vi "一体站流程自动启动.vi"(11 "参数":T1) -> ()   [LabVIEW 2016, in "PLC.lvlib"]
uses:
  PLC.lvlib
panel:
  out "s? t:f":enum16{"初始化", "采配水启动", "仪器操作", "反冲洗", "结束"}(ring)
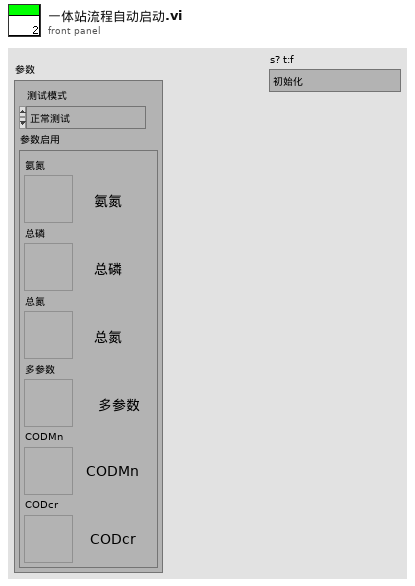
[diagram p1: front panel]
types:
  T1 = cluster{"测试模式":enum16{"正常测试", "集成干预"}, "参数启用":cluster{"氨氮":bool, "总磷":bool, "总氮":bool, "多参数":bool, "CODMn":bool, "CODcr":bool}}
  T2 = cluster{"命令":string, cluster{"starting address":u16, "holding register value":u16}}
  T3 = enum16{"启动测量", "标样核查", "零点核查", "跨度核查", "空白测试", "平行样测试", "加标回收", "空白校准", "标样校准", "初始化（清洗）", "停止测试", "仪器重启", "校时", "模式设置", "测量间隔设置"}
  T4 = cluster{"时间标识":timestamp, "设备":string, "日志信息":string, "流程参数":string}
  T5 = cluster{"测量模式":enum16{"水样测量", "标样核查", "零点核查", "跨度核查", "空白测试", "加标回收", "平行样", "校零", "校标"}}
  T6 = cluster{"时间标识":timestamp, "设备":string, "日志信息":string}
  T7 = enum16{"空闲", "水样测试", "标样核查", "零点核查", "跨度核查", "空白测试", "平行样测试", "加标回收", "空白校准", "标样校准", "初始化（清洗）"}
  T8 = cluster{"R0":i16, "R1":i16, "R2":i16, "R3":i16, "R4":i16, "R5":i16, "R6":i16, "R7":i16, "R8":i16, "R9":i16, "R10":i16, "R11":i16, "R12":i16, "R13":i16, "R14":i16, "R15":i16, "R16":i16, "R17":i16, "R18":i16, "R19":i16, "R20":i16, "R21":i16, "R22":i16, "R23":i16, "R24":i16, "R25":i16, "R26":i16, "R27":i16, "R28":i16, "R29":i16, "R30":i16, "R31":i16, "R32":i16, "R33":i16, "R34":i16, "R35":i16, "R36":i16, "R37":i16, "R38":i16, "R39":i16, "R40":i16, "R41":i16, "R42":i16, "R43":i16, "R44":i16, "R45":i16, "R46":i16, "R47":i16, "R48":i16, "R49":i16, "R50":i16, "R51":i16, "R52":i16, "R53":i16, "R54":i16, "R55":i16, "R56":i16}
  T9 = cluster{"R100":i16, "R101":i16, "R102":i16, "R103":i16, "R104":i16, "R105":i16, "R106":i16, "R107":i16, "R108":i16, "R109":i16, "R110":i16, "R111":i16, "R112":i16, "R113":i16, "R114":i16, "R115":i16, "R116":i16, "R117":i16, "R118":i16, "R119":i16, "R120":i16, "R121":i16, "R122":i16, "R123":i16}
  T10 = enum32{"Bad", "Idle", "Run top level", "Running"}
  T11 = cluster{"水样测试量程模式":enum16{"H", "L", "AUTO"}, "空白核查量程模式":enum16{"H", "L", "AUTO"}, "跨度核查量程模式":enum16{"H", "L", "AUTO"}}
  T12 = cluster{"氨氮":bool, "总磷":bool, "总氮":bool, "多参数":bool, "CODMn":bool, "CODcr":bool}
  T13 = cluster{"时间标识":timestamp, "参数":string, "集成干预测试浓度值":dbl, "集成干预前测试时间":timestamp, "集成干预前测试浓度值":dbl}
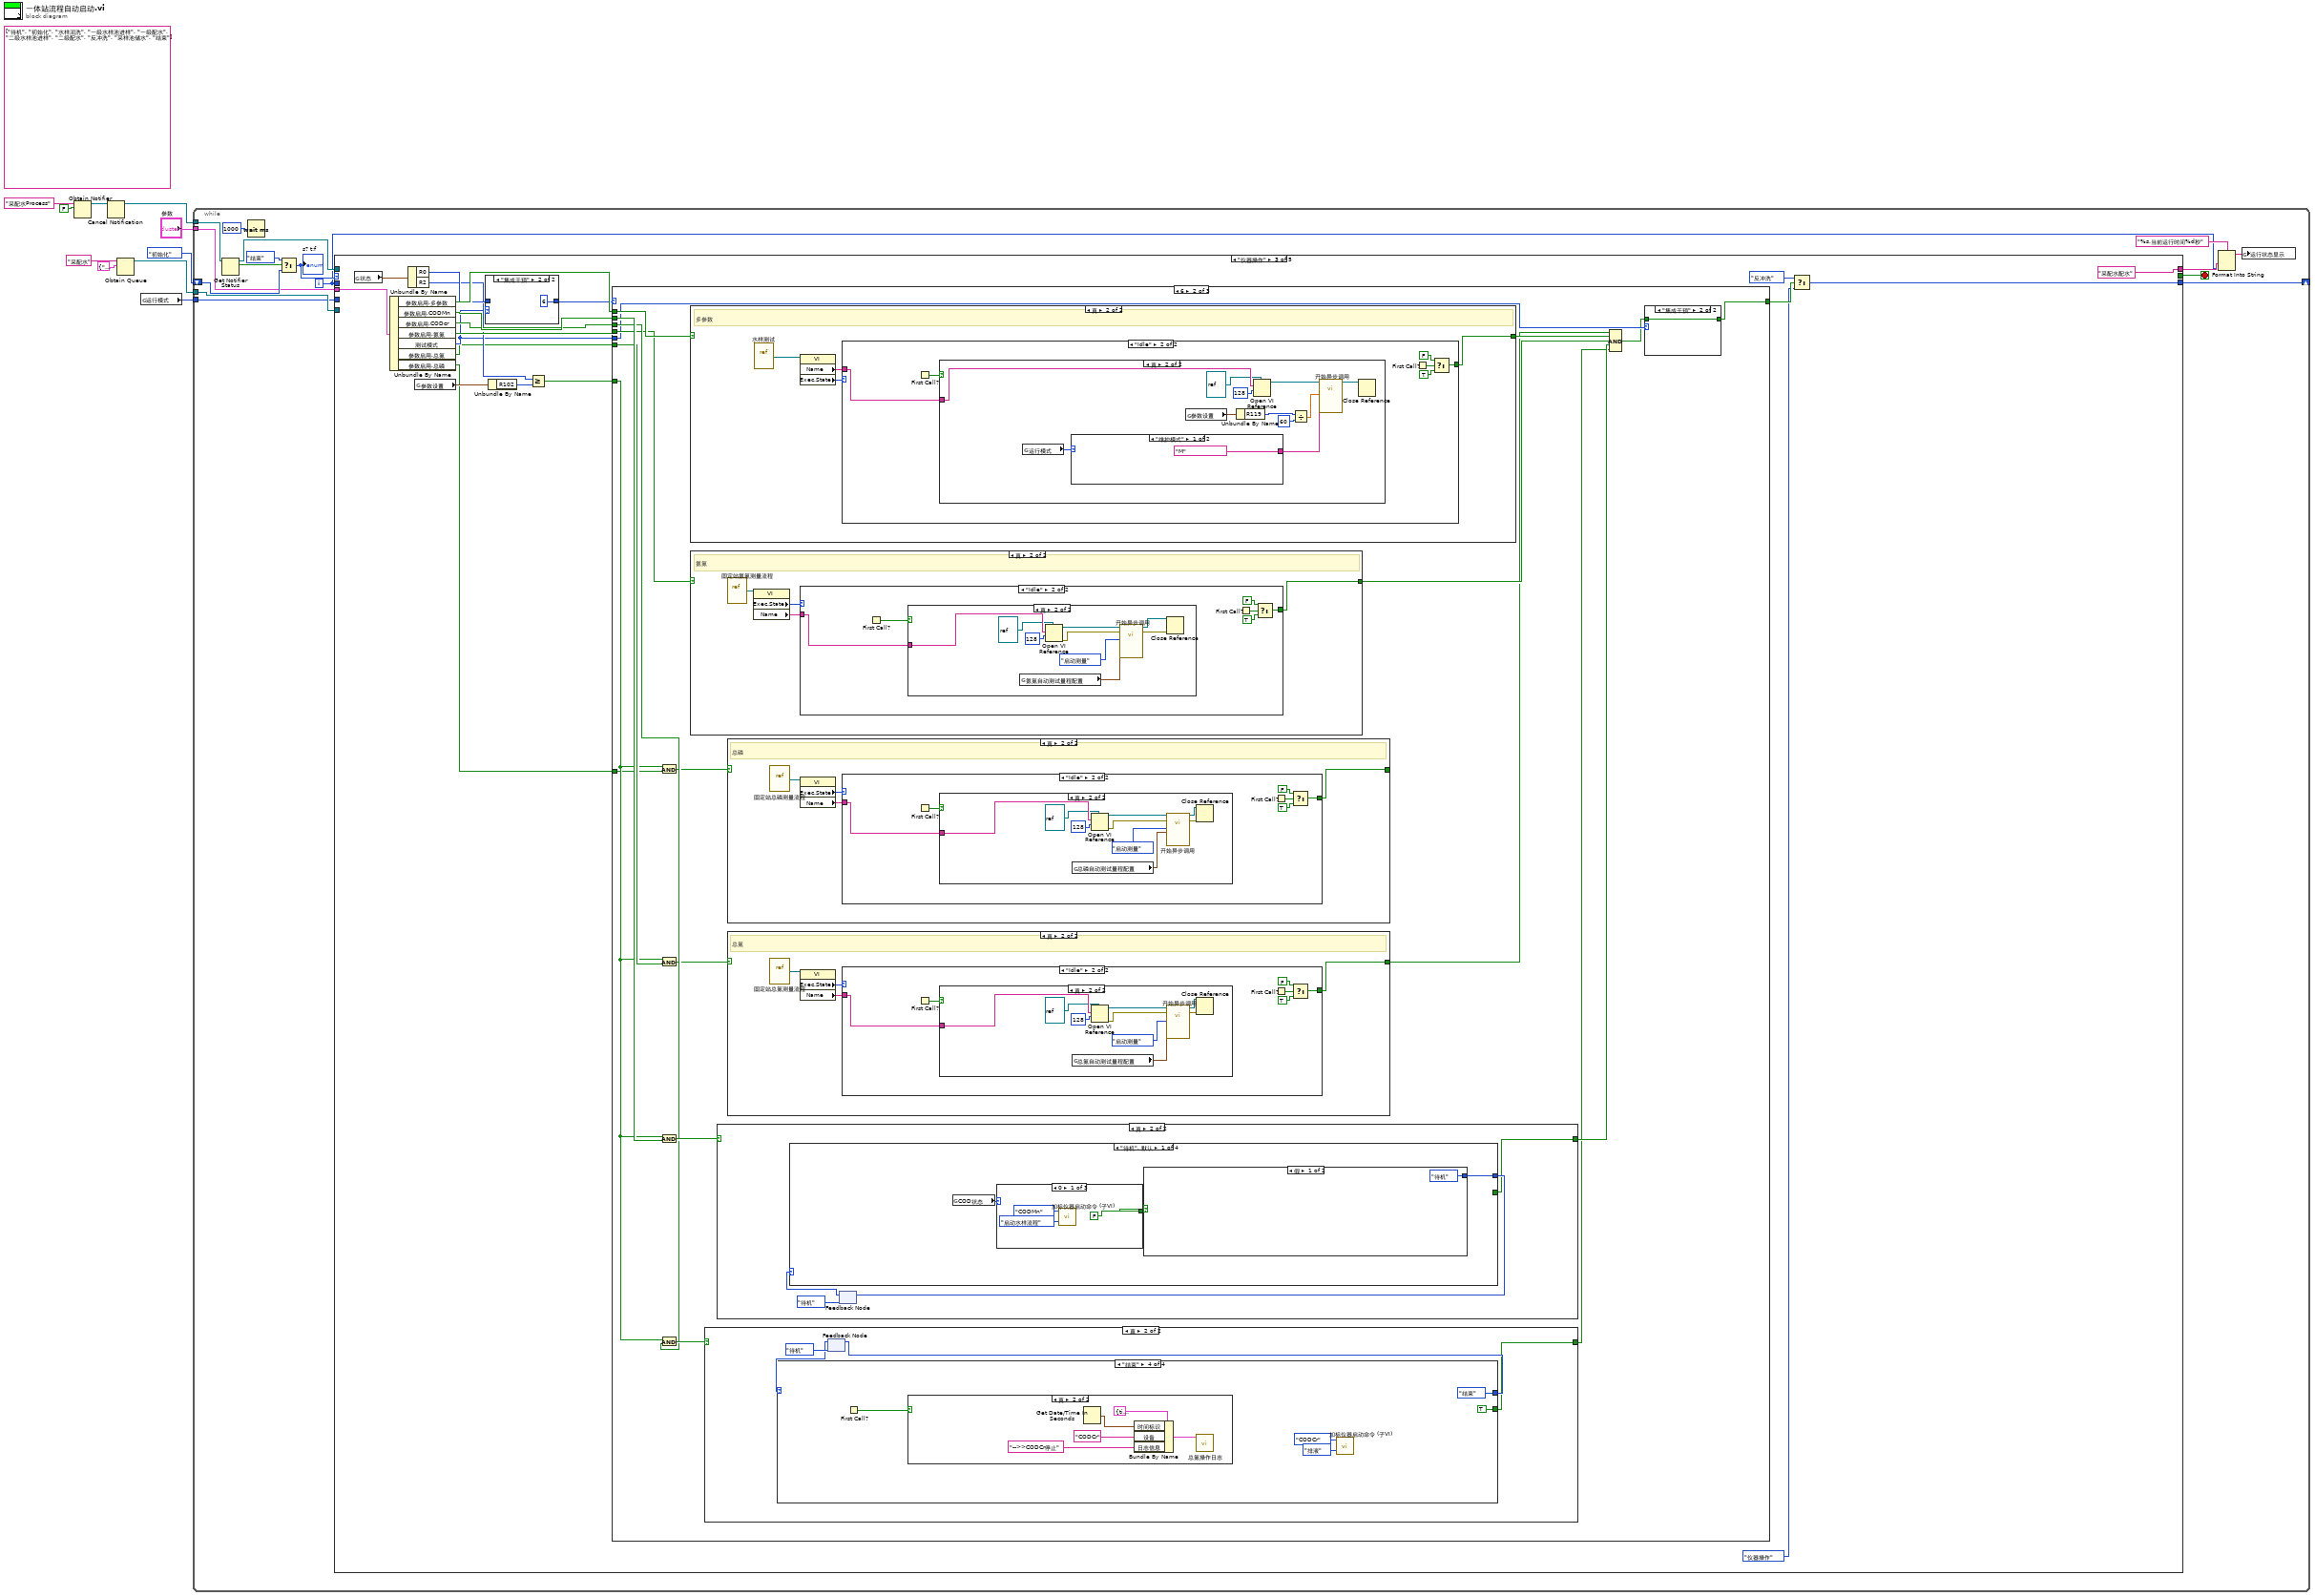
[diagram p0: block diagram]
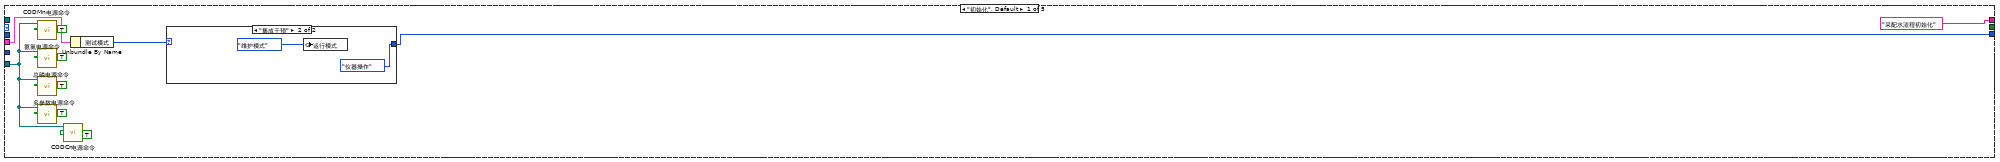
[diagram p2: hidden frame]
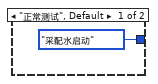
[diagram p3: hidden frame]
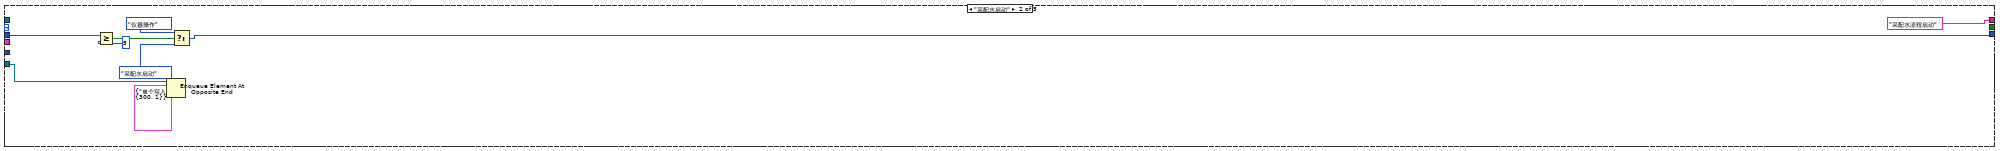
[diagram p4: hidden frame]
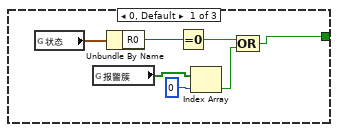
[diagram p6: hidden frame]
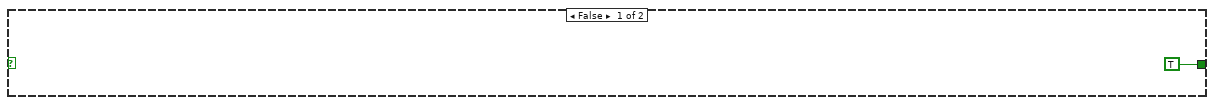
[diagram p7: hidden frame]
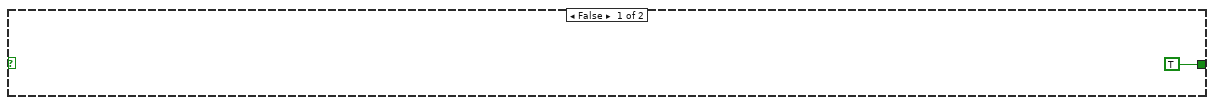
[diagram p10: hidden frame]
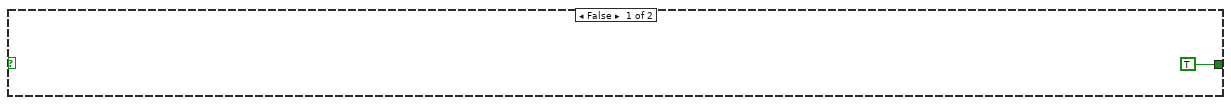
[diagram p14: hidden frame]
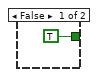
[diagram p17: hidden frame]
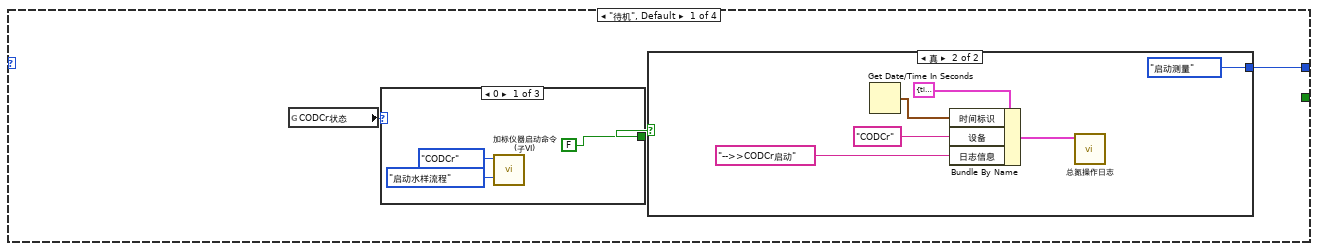
[diagram p18: hidden frame]
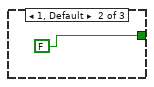
[diagram p19: hidden frame]
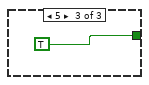
[diagram p20: hidden frame]
diagram:
  (unwired) string[][] [["待机"], ["初始化"], ["水样润洗"], ["一级水样池进样"], ["一级配水"], ["二级水样池进样"], ["二级配水"], ["反冲洗"], ["采样池储水"], ["结束"]] ("项名")
  n1 = Obtain Notifier(name (unnamed)="采配水Process" ("名称（未命名）"), notification data type=FALSE) -> (notifier out=w4:refnum<notifier>)  [unwired: 2 in, 2 out]
  n2 = Cancel Notification(0:w4) -> (8:w3:refnum<notifier>)  [unwired: 1 in, 2 out]
  n3 = Obtain Queue(name (unnamed)="采配水" ("名称（未命名）"), element data type=cluster{"命令":string, "数据":variant} {"命令"="", "数据"=variant}) -> (queue out=w7:refnum<queue>)  [unwired: 3 in, 2 out]
  n4 = global read "系统设置全局变量.vi" "运行模式"() -> (w1:enum16{"维护模式", "常规模式", "应急模式", "质控模式"})
  n5 = while {
    shift-right: [w23] -> _
    shift-left: enum16{"初始化", "采配水启动", "仪器操作", "反冲洗", "结束"}."初始化" ("枚举") -> [w19]
    tunnel: w7 -> [w26]
    tunnel: w3 -> [w22]
    tunnel: "参数" -> [w13]
    tunnel: w1 -> [w12]
    i -> [w11]
    stop <- w25 stop-if-true
    n6 = Get Notifier Status(notifier=w22) -> (notifier out=w14:refnum<notifier>, current notification=w21:bool)  [unwired: 1 in, 3 out]
    n7 = Wait (ms)(milliseconds to wait=u32 1000 ("等待时间（毫秒）")) -> ()  [unwired: 1 out]
    n8 = Select(t=enum16{"初始化", "采配水启动", "仪器操作", "反冲洗", "结束"}."结束" ("枚举"), s=w21, f=w19) -> (s? t:f=w18:enum16{"初始化", "采配水启动", "仪器操作", "反冲洗", "结束"})
    "s? t:f" <- w18
    n9 = case shown="\"仪器操作\"" w18 {
      tunnel: w26 -> [w31 w48 _ _ w479]
      tunnel: [_ _ _ _ TRUE] -> w25
      tunnel: [w30 w40 w63 w311 enum16{"初始化", "采配水启动", "仪器操作", "反冲洗", "结束"}."结束" ("枚举")] -> w23
      tunnel: ["采配水流程初始化" "采配水流程启动" "采配水配水" "等待测试完成" "采配水结束"] -> w15
      tunnel: w14 -> [_ _ _ _ w480]
      tunnel: w13 -> [w28 _ w66 w310 w476]
      tunnel: w12 -> [_ _ _ _ w475]
      tunnel: w11 -> [_ w46 _ _ _]
      frame "初始化", Default {
        n10 = call "CODMn电源命令.vi"("通电/断电"=TRUE, "队列"=w31) -> ()  [unwired: 9 in, 1 out]
        n11 = call "氨氮电源命令.vi"("通电/断电"=TRUE, "队列"=w31) -> ()  [unwired: 9 in, 1 out]
        n12 = call "总磷电源命令.vi"("通电/断电"=TRUE, "队列"=w31) -> ()  [unwired: 9 in, 1 out]
        n13 = call "多参数电源命令.vi"("通电/断电"=TRUE, "队列"=w31) -> ()  [unwired: 9 in, 1 out]
        n14 = call "CODCr电源命令.vi"("通电/断电"=TRUE, "队列"=w31) -> ()  [unwired: 9 in, 1 out]
        n15 = Unbundle By Name(w28) -> ("测试模式"=w27:enum16{"正常测试", "集成干预"})
        n16 = case shown="\"集成干预\"" w27 {
          tunnel: [enum16{"初始化", "采配水启动", "仪器操作", "反冲洗", "结束"}."采配水启动" ("枚举") enum16{"初始化", "采配水启动", "仪器操作", "反冲洗", "结束"}."仪器操作" ("枚举")] -> w30
          frame "正常测试", Default {
          }
          frame "集成干预" {
            n17 = global write "系统设置全局变量.vi" "运行模式"(enum16{"维护模式", "常规模式", "应急模式", "质控模式"}."维护模式" ("运行模式")) -> ()
          }
        }
      }
      frame "采配水启动" {
        n18 = Greater Or Equal?(x=w46, y=5) -> (x >= y?=w43:bool)
        n19 = Enqueue Element At Opposite End(queue=w48, element=T2 {"命令"="单个写入", {"starting address"=300, "holding register value"=1}} ("元素")) -> ()  [unwired: 2 in, 3 out]
        n20 = Select(t=enum16{"初始化", "采配水启动", "仪器操作", "反冲洗", "结束"}."仪器操作" ("枚举"), s=w43, f=enum16{"初始化", "采配水启动", "仪器操作", "反冲洗", "结束"}."采配水启动" ("枚举")) -> (s? t:f=w40:enum16{"初始化", "采配水启动", "仪器操作", "反冲洗", "结束"})
      }
      frame "仪器操作" {
        n21 = global read "采配水全局变量.vi" "状态"() -> (w68:T8)
        n22 = Unbundle By Name(w66) -> ("参数启用.多参数"=w61:bool, "参数启用.CODMn"=w60:bool, "参数启用.CODcr"=w59:bool, "参数启用.氨氮"=w58:bool, "测试模式"=w51:enum16{"正常测试", "集成干预"}, "参数启用.总氮"=w50:bool, "参数启用.总磷"=w49:bool)
        n23 = Unbundle By Name(w68) -> ("R0"=w57:i16, "R2"=w52:i16)
        n24 = global read "采配水全局变量.vi" "参数设置"() -> (w54:T9)
        n25 = case shown="\"集成干预\"" w51 {
          tunnel: w57 -> [w69 _]
          tunnel: [w69 i16 6 ("R0")] -> w56
          frame "正常测试", Default {
          }
          frame "集成干预" {
          }
        }
        n26 = Unbundle By Name(w54) -> ("R102"=w55:i16)
        n27 = Greater Or Equal?(x=w52, y=w55) -> (x >= y?=w53:bool)
        n28 = case shown="6" w56 {
          tunnel: [w72 w84 TRUE] -> w65
          tunnel: w61 -> [_ w96 _]
          tunnel: w60 -> [_ w95 _]
          tunnel: w59 -> [_ w92 _]
          tunnel: w58 -> [_ w91 _]
          tunnel: w53 -> [_ w80 _]
          tunnel: w51 -> [_ w86 _]
          tunnel: w50 -> [_ w83 _]
          tunnel: w49 -> [_ w79 _]
          frame 0, Default {
            n29 = global read "采配水全局变量.vi" "状态"() -> (w75:T8)
            n30 = global read "采配水全局变量.vi" "报警簇"() -> (w76:bool[])
            n31 = Unbundle By Name(w75) -> ("R0"=w74:i16)
            n32 = Equal To 0?(x=w74) -> (x = 0?=w77:bool)
            n33 = Index Array(array=w76, index=0 ("索引")) -> (element=w71:bool)
            n34 = Compound Arithmetic op=OR ("复合运算")(w77, w71) -> (w72:bool)
          }
          frame 6 {
            n35 = And(x=w80, y=w79) -> (x .and. y?=w78:bool)
            n36 = And(x=w80, y=w83) -> (x .and. y?=w82:bool)
            n37 = And(x=w80, y=w95) -> (x .and. y?=w94:bool)
            n38 = And(x=w80, y=w92) -> (x .and. y?=w93:bool)
            n39 = case shown="真" w96 {
              tunnel: [TRUE ("t") w284] -> w90
              frame False {
              }
              frame True {
                # "多参数"
                n40 = vi-ref "水样测试.vi"() -> (w286:refnum<vi>)
                n41 = property class="VI"(reference=w286) -> ("Name"=w285:string, "Exec.State"=w287:T10)  [unwired: 1 in, 2 out]
                n42 = case shown="\"Idle\"" w287 {
                  tunnel: w285 -> [_ w293]
                  tunnel: [_ w288] -> w284
                  frame "Bad", Default {
                  }
                  frame "Idle" {
                    n43 = First Call?() -> (First Call?: T/F=w292:bool)
                    n44 = case shown="真" w292 {
                      tunnel: w293 -> [_ w303]
                      frame False {
                      }
                      frame True {
                        n45 = global read "系统设置全局变量.vi" "运行模式"() -> (w300:enum16{"维护模式", "常规模式", "应急模式", "质控模式"})
                        n46 = case shown="\"维护模式\"" w300 {
                          tunnel: ["M" ("数据标记表") "N" ("数据标记表")] -> w295
                          frame "维护模式" {
                          }
                          frame "常规模式", Default {
                          }
                        }
                        n47 = global read "采配水全局变量.vi" "参数设置"() -> (w299:T9)
                        n48 = Unbundle By Name(w299) -> ("R119"=w298:i16)
                        n49 = Open VI Reference(type specifier VI Refnum (for type only)=refnum<vi> refnum, vi path=w303, options=128 ("选项")) -> (vi reference=w302:refnum<vi>)  [unwired: 3 in, 1 out]
                        n50 = Divide(x=w298, y=i16 60) -> (x/y=w296:dbl)
                        n51 = call-by-ref "开始异步调用"(reference=w302, "数据标记表"=w295, "水样测试时间"=w296) -> (reference out=w301:refnum<vi>)  [unwired: 11 in, 1 out]
                        n52 = Close Reference(reference=w301) -> ()  [unwired: 1 in, 1 out]
                      }
                    }
                    n53 = First Call?() -> (First Call?: T/F=w291:bool)
                    n54 = Select(t=FALSE, s=w291, f=TRUE) -> (s? t:f=w288:bool)
                  }
                }
              }
            }
            n55 = case "条件结构" shown="真" w91 {
              tunnel: [TRUE ("t") w139] -> w89
              frame False {
              }
              frame True {
                # "氨氮"
                n56 = vi-ref "固定站氨氮测量流程.vi"() -> (w142:refnum<vi>)
                n57 = property class="VI"(reference=w142) -> ("Exec.State"=w141:T10, "Name"=w140:string)  [unwired: 1 in, 2 out]
                n58 = case shown="\"Idle\"" w141 {
                  tunnel: w140 -> [_ w148]
                  tunnel: [_ w143] -> w139
                  frame "Bad", Default {
                  }
                  frame "Idle" {
                    n59 = First Call?() -> (First Call?: T/F=w147:bool)
                    n60 = case shown="真" w147 {
                      tunnel: w148 -> [_ w154]
                      frame False {
                      }
                      frame True {
                        n61 = global read "氨氮断电保存全局变量.vi" "氨氮自动测试量程配置"() -> (w151:T11)
                        n62 = Open VI Reference(type specifier VI Refnum (for type only)=refnum<vi> refnum, vi path=w154, options=128 ("选项")) -> (vi reference=w152:refnum<vi>, error out=w155:errorcluster)  [unwired: 3 in]
                        n63 = call-by-ref "开始异步调用"(reference=w152, error in=w155, "总磷量程模式"=w151, "控制命令"=T3."启动测量") -> (reference out=w156:refnum<vi>, error out=w157:errorcluster)  [unwired: 10 in]
                        n64 = Close Reference(reference=w156, error in (no error)=w157) -> ()  [unwired: 1 out]
                      }
                    }
                    n65 = First Call?() -> (First Call?: T/F=w146:bool)
                    n66 = Select(t=FALSE, s=w146, f=TRUE) -> (s? t:f=w143:bool)
                  }
                }
              }
            }
            n67 = case shown="真" w93 {
              tunnel: [TRUE w159] -> w87
              frame False {
              }
              frame True {
                n68 = feedback #1(enum16{"待机", "启动测量", "测量中", "结束"}."待机") -> (w161:enum16{"待机", "启动测量", "测量中", "结束"})
                n69 = case shown="\"结束\"" w161 {
                  tunnel: [w165 w186 w206 enum16{"待机", "启动测量", "测量中", "结束"}."结束"] -> w160
                  tunnel: [_ _ _ TRUE] -> w159
                  frame "待机", Default {
                    n70 = global read "加标回收状态全局变量.vi" "CODCr状态"() -> (w164:u16)
                    n71 = case shown="0" w164 {
                      tunnel: [FALSE ("s") FALSE ("s") TRUE ("s")] -> w163
                      frame 0 {
                        n72 = call "加标仪器启动命令 (子VI).vi"("启动命令"=enum16{"启动水样流程", "启动加标流程", "排液", "停止", "柱塞泵启动"}."启动水样流程", "仪器"=enum16{"", "氨氮", "总磷", "总氮", "CODMn", "CODCr"}."CODCr") -> ()  [unwired: 9 in, 1 out]
                      }
                      frame 1, Default {
                      }
                      frame 5 {
                      }
                    }
                    n73 = case shown="真" w163 {
                      tunnel: [enum16{"待机", "启动测量", "测量中", "结束"}."待机" enum16{"待机", "启动测量", "测量中", "结束"}."启动测量"] -> w165
                      frame False {
                      }
                      frame True {
                        n74 = Get Date/Time In Seconds() -> (seconds since 1Jan1904=w176:timestamp)
                        n75 = Bundle By Name(cluster=T4 {"时间标识"=timestamp(0 s since 1904-01-01), "设备"="", "日志信息"="", "流程参数"=""} ("data in"), "时间标识"=w176, "设备"="CODCr", "日志信息"="-->>CODCr启动") -> (w172:T4)
                        n76 = call "总氮操作日志.vi"("data in"=w172) -> ()  [unwired: 11 in]
                      }
                    }
                  }
                  frame "启动测量" {
                    # "CODcr"
                    n77 = feedback #2() -> (w182:i32)  [unwired: 1 in]
                    n78 = Increment(x=w182) -> (x+1=w183:i32)
                    n79 = First Call?() -> (First Call?: T/F=w181:bool)
                    n80 = call "CODCr启动命令 (子VI).vi"("启动测量模式"=T5 {"测量模式"=enum."水样测量"}) -> ()  [unwired: 11 in]
                    n81 = Select(t=0, s=w181, f=w183) -> (s? t:f=w184:i32)
                    n82 = feedback-in #2(w184) -> ()
                    n83 = Greater Or Equal?(x=w184, y=60) -> (x >= y?=w179:bool)
                    n84 = case shown="真" w179 {
                      tunnel: [w187 enum16{"待机", "启动测量", "测量中", "结束"}."结束"] -> w186
                      frame False {
                        n85 = global read "CODcr全局变量.vi" "工作状态"() -> (w188:T7)
                        n86 = Not Equal To 0?(x=w188) -> (x != 0?=w189:bool)
                        n87 = Select(t=enum16{"待机", "启动测量", "测量中", "结束"}."测量中", s=w189, f=enum16{"待机", "启动测量", "测量中", "结束"}."启动测量") -> (s? t:f=w187:enum16{"待机", "启动测量", "测量中", "结束"})
                      }
                      frame True {
                        n88 = Get Date/Time In Seconds() -> (seconds since 1Jan1904=w198:timestamp)
                        n89 = Bundle By Name(cluster=T6 {"时间标识"=timestamp(0 s since 1904-01-01), "设备"="", "日志信息"=""} ("data in"), "时间标识"=w198, "设备"="CODCr", "日志信息"="CODCr启动失败") -> (w192:T6)
                        n90 = call "报警信息字段定义.vi"("table输入"="报警信息", "data in"=w192) -> ("table输出"=w195:string, "columns"=w196:string[], "data out"=w197:T6)  [unwired: 7 in]
                        n91 = call "插入数据.vi"("data"=w197, "columns"=w196, "database"="database3.mdb", "table"=w195) -> ()  [unwired: 7 in, 1 out]
                      }
                    }
                  }
                  frame "测量中" {
                    n92 = global read "CODcr全局变量.vi" "工作状态"() -> (w205:T7)
                    n93 = Equal?(x=w205, y=T7."空闲" ("工作状态")) -> (x = y?=w204:bool)
                    n94 = case shown="假" w204 {
                      tunnel: [w207 enum16{"待机", "启动测量", "测量中", "结束"}."结束"] -> w206
                      frame False {
                        n95 = flat-sequence {
                          tunnel: [enum16{"待机", "启动测量", "测量中", "结束"}."测量中"] -> w207
                          frame #0 {
                            n96 = Wait (ms)(milliseconds to wait=u32 1000 ("等待时间（毫秒）")) -> ()  [unwired: 1 out]
                          }
                          frame #1 {
                          }
                        }
                      }
                      frame True {
                      }
                    }
                  }
                  frame "结束" {
                    n97 = First Call?() -> (First Call?: T/F=w213:bool)
                    n98 = case shown="真" w213 {
                      frame False {
                      }
                      frame True {
                        n99 = Get Date/Time In Seconds() -> (seconds since 1Jan1904=w220:timestamp)
                        n100 = Bundle By Name(cluster=T4 {"时间标识"=timestamp(0 s since 1904-01-01), "设备"="", "日志信息"="", "流程参数"=""} ("data in"), "时间标识"=w220, "设备"="CODCr", "日志信息"="-->>CODCr停止") -> (w216:T4)
                        n101 = call "总氮操作日志.vi"("data in"=w216) -> ()  [unwired: 11 in]
                      }
                    }
                    n102 = call "加标仪器启动命令 (子VI).vi"("启动命令"=enum16{"启动水样流程", "启动加标流程", "排液", "停止", "柱塞泵启动"}."排液", "仪器"=enum16{"", "氨氮", "总磷", "总氮", "CODMn", "CODCr"}."CODCr") -> ()  [unwired: 9 in, 1 out]
                  }
                }
                n103 = feedback-in #1(w160) -> ()
              }
            }
            n104 = case shown="真" w94 {
              tunnel: [TRUE w222] -> w88
              frame False {
              }
              frame True {
                n105 = feedback #3(enum16{"待机", "启动测量", "测量中", "结束"}."待机") -> (w224:enum16{"待机", "启动测量", "测量中", "结束"})
                n106 = case shown="\"待机\", 默认" w224 {
                  tunnel: [w228 w249 w268 enum16{"待机", "启动测量", "测量中", "结束"}."结束"] -> w223
                  tunnel: [_ _ _ TRUE] -> w222
                  frame "待机", Default {
                    n107 = global read "加标回收状态全局变量.vi" "COD状态"() -> (w227:u16)
                    n108 = case shown="0" w227 {
                      tunnel: [FALSE ("s") FALSE ("s") TRUE ("s")] -> w226
                      frame 0 {
                        n109 = call "加标仪器启动命令 (子VI).vi"("启动命令"=enum16{"启动水样流程", "启动加标流程", "排液", "停止", "柱塞泵启动"}."启动水样流程", "仪器"=enum16{"", "氨氮", "总磷", "总氮", "CODMn", "CODCr"}."CODMn") -> ()  [unwired: 9 in, 1 out]
                      }
                      frame 1, Default {
                      }
                      frame 5 {
                      }
                    }
                    n110 = case shown="假" w226 {
                      tunnel: [enum16{"待机", "启动测量", "测量中", "结束"}."待机" enum16{"待机", "启动测量", "测量中", "结束"}."启动测量"] -> w228
                      frame False {
                      }
                      frame True {
                        n111 = Get Date/Time In Seconds() -> (seconds since 1Jan1904=w239:timestamp)
                        n112 = Bundle By Name(cluster=T4 {"时间标识"=timestamp(0 s since 1904-01-01), "设备"="", "日志信息"="", "流程参数"=""} ("data in"), "时间标识"=w239, "设备"="CODMn", "日志信息"="-->>CODMn启动") -> (w235:T4)
                        n113 = call "总氮操作日志.vi"("data in"=w235) -> ()  [unwired: 11 in]
                      }
                    }
                  }
                  frame "启动测量" {
                    # "CODMn"
                    n114 = feedback #4() -> (w245:i32)  [unwired: 1 in]
                    n115 = Increment(x=w245) -> (x+1=w246:i32)
                    n116 = First Call?() -> (First Call?: T/F=w244:bool)
                    n117 = call "CODMn启动命令 (子VI).vi"("启动测量模式"=T5 {"测量模式"=enum."水样测量"}) -> ()  [unwired: 11 in]
                    n118 = Select(t=0, s=w244, f=w246) -> (s? t:f=w247:i32)
                    n119 = feedback-in #4(w247) -> ()
                    n120 = Greater Or Equal?(x=w247, y=60) -> (x >= y?=w242:bool)
                    n121 = case shown="假" w242 {
                      tunnel: [w251 enum16{"待机", "启动测量", "测量中", "结束"}."结束"] -> w249
                      frame False {
                        n122 = global read "运行时序全局变量.vi" "多列列表框"() -> (w250:i32)
                        n123 = Not Equal To 0?(x=w250) -> (x != 0?=w252:bool)
                        n124 = Select(t=enum16{"待机", "启动测量", "测量中", "结束"}."测量中", s=w252, f=enum16{"待机", "启动测量", "测量中", "结束"}."启动测量") -> (s? t:f=w251:enum16{"待机", "启动测量", "测量中", "结束"})
                      }
                      frame True {
                        n125 = Get Date/Time In Seconds() -> (seconds since 1Jan1904=w261:timestamp)
                        n126 = Bundle By Name(cluster=T6 {"时间标识"=timestamp(0 s since 1904-01-01), "设备"="", "日志信息"=""} ("data in"), "时间标识"=w261, "设备"="CODMn", "日志信息"="CODMn启动失败") -> (w255:T6)
                        n127 = call "报警信息字段定义.vi"("table输入"="报警信息", "data in"=w255) -> ("table输出"=w258:string, "columns"=w259:string[], "data out"=w260:T6)  [unwired: 7 in]
                        n128 = call "插入数据.vi"("data"=w260, "columns"=w259, "database"="database3.mdb", "table"=w258) -> ()  [unwired: 7 in, 1 out]
                      }
                    }
                  }
                  frame "测量中" {
                    n129 = global read "运行时序全局变量.vi" "多列列表框"() -> (w267:i32)
                    n130 = Equal To 0?(x=w267) -> (x = 0?=w266:bool)
                    n131 = case shown="假" w266 {
                      tunnel: [w269 enum16{"待机", "启动测量", "测量中", "结束"}."结束"] -> w268
                      frame False {
                        n132 = flat-sequence {
                          tunnel: [enum16{"待机", "启动测量", "测量中", "结束"}."测量中"] -> w269
                          frame #0 {
                            n133 = Wait (ms)(milliseconds to wait=u32 1000 ("等待时间（毫秒）")) -> ()  [unwired: 1 out]
                          }
                          frame #1 {
                          }
                        }
                      }
                      frame True {
                      }
                    }
                  }
                  frame "结束" {
                    n134 = call "加标仪器启动命令 (子VI).vi"("启动命令"=enum16{"启动水样流程", "启动加标流程", "排液", "停止", "柱塞泵启动"}."排液", "仪器"=enum16{"", "氨氮", "总磷", "总氮", "CODMn", "CODCr"}."CODMn") -> ()  [unwired: 9 in, 1 out]
                    n135 = First Call?() -> (First Call?: T/F=w275:bool)
                    n136 = case shown="真" w275 {
                      frame False {
                      }
                      frame True {
                        n137 = Get Date/Time In Seconds() -> (seconds since 1Jan1904=w282:timestamp)
                        n138 = Bundle By Name(cluster=T4 {"时间标识"=timestamp(0 s since 1904-01-01), "设备"="", "日志信息"="", "流程参数"=""} ("data in"), "时间标识"=w282, "设备"="CODMn", "日志信息"="-->>CODMn停止") -> (w278:T4)
                        n139 = call "总氮操作日志.vi"("data in"=w278) -> ()  [unwired: 11 in]
                      }
                    }
                  }
                }
                n140 = feedback-in #3(w223) -> ()
              }
            }
            n141 = case "条件结构" shown="真" w78 {
              tunnel: [TRUE ("t") w98] -> _
              frame False {
              }
              frame True {
                # "总磷"
                n142 = vi-ref "固定站总磷测量流程.vi"() -> (w101:refnum<vi>)
                n143 = property class="VI"(reference=w101) -> ("Exec.State"=w100:T10, "Name"=w99:string)  [unwired: 1 in, 2 out]
                n144 = case shown="\"Idle\"" w100 {
                  tunnel: w99 -> [_ w107]
                  tunnel: [_ w102] -> w98
                  frame "Bad", Default {
                  }
                  frame "Idle" {
                    n145 = First Call?() -> (First Call?: T/F=w106:bool)
                    n146 = case shown="真" w106 {
                      tunnel: w107 -> [_ w113]
                      frame False {
                      }
                      frame True {
                        n147 = global read "总磷断电保存全局变量.vi" "总磷自动测试量程配置"() -> (w108:T11)
                        n148 = Open VI Reference(type specifier VI Refnum (for type only)=refnum<vi> refnum, vi path=w113, options=128 ("选项")) -> (vi reference=w111:refnum<vi>, error out=w114:errorcluster)  [unwired: 3 in]
                        n149 = call-by-ref "开始异步调用"(reference=w111, error in=w114, "总磷量程模式"=w108, "控制命令"=T3."启动测量") -> (reference out=w115:refnum<vi>, error out=w116:errorcluster)  [unwired: 10 in]
                        n150 = Close Reference(reference=w115, error in (no error)=w116) -> ()  [unwired: 1 out]
                      }
                    }
                    n151 = First Call?() -> (First Call?: T/F=w105:bool)
                    n152 = Select(t=FALSE, s=w105, f=TRUE) -> (s? t:f=w102:bool)
                  }
                }
              }
            }
            n153 = case "条件结构" shown="真" w82 {
              tunnel: [TRUE ("t") w118] -> w81
              frame False {
              }
              frame True {
                # "总氮"
                n154 = vi-ref "固定站总氮测量流程.vi"() -> (w121:refnum<vi>)
                n155 = property class="VI"(reference=w121) -> ("Exec.State"=w120:T10, "Name"=w119:string)  [unwired: 1 in, 2 out]
                n156 = case shown="\"Idle\"" w120 {
                  tunnel: w119 -> [_ w127]
                  tunnel: [_ w122] -> w118
                  frame "Bad", Default {
                  }
                  frame "Idle" {
                    n157 = First Call?() -> (First Call?: T/F=w126:bool)
                    n158 = case shown="真" w126 {
                      tunnel: w127 -> [_ w133]
                      frame False {
                      }
                      frame True {
                        n159 = global read "总氮断电保存全局变量.vi" "总氮自动测试量程配置"() -> (w130:T11)
                        n160 = Open VI Reference(type specifier VI Refnum (for type only)=refnum<vi> refnum, vi path=w133, options=128 ("选项")) -> (vi reference=w131:refnum<vi>, error out=w134:errorcluster)  [unwired: 3 in]
                        n161 = call-by-ref "开始异步调用"(reference=w131, error in=w134, "总磷量程模式"=w130, "控制命令"=T3."启动测量") -> (reference out=w135:refnum<vi>, error out=w136:errorcluster)  [unwired: 10 in]
                        n162 = Close Reference(reference=w135, error in (no error)=w136) -> ()  [unwired: 1 out]
                      }
                    }
                    n163 = First Call?() -> (First Call?: T/F=w125:bool)
                    n164 = Select(t=FALSE, s=w125, f=TRUE) -> (s? t:f=w122:bool)
                  }
                }
              }
            }
            n165 = Compound Arithmetic op=AND ("复合运算")(w81, w90, w89, w88, w87) -> (w85:bool)
            n166 = case shown="\"集成干预\"" w86 {
              tunnel: w85 -> [_ w137]
              tunnel: [_ w137] -> w84
              frame "正常测试", Default {
              }
              frame "集成干预" {
              }
            }
          }
          frame 7..9 {
          }
        }
        n167 = Select(t=enum16{"初始化", "采配水启动", "仪器操作", "反冲洗", "结束"}."反冲洗" ("枚举"), s=w65, f=enum16{"初始化", "采配水启动", "仪器操作", "反冲洗", "结束"}."仪器操作" ("枚举")) -> (s? t:f=w63:enum16{"初始化", "采配水启动", "仪器操作", "反冲洗", "结束"})
      }
      frame "反冲洗" {
        n168 = First Call?() -> (First Call?: T/F=w308:bool)
        n169 = case shown="真" w308 {
          tunnel: w310 -> [_ w319]
          frame False {
          }
          frame True {
            n170 = Unbundle By Name(w319) -> ("测试模式"=w318:enum16{"正常测试", "集成干预"}, "参数启用"=w317:T12)
            n171 = case shown="\"正常测试\", 默认" w318 {
              tunnel: w317 -> [w322 w408]
              frame "正常测试", Default {
                n172 = global read "系统设置全局变量.vi" "运行模式"() -> (w320:enum16{"维护模式", "常规模式", "应急模式", "质控模式"})
                n173 = global read "采配水全局变量.vi" "报警簇"() -> (w327:bool[])
                n174 = case shown="\"维护模式\"" w320 {
                  tunnel: ["M" ("table") "N" ("table")] -> w321
                  frame "维护模式" {
                  }
                  frame "常规模式", Default {
                  }
                }
                n175 = Index Array(array=w327, index #1=0 ("索引"), index #2=11 ("索引")) -> (element #1=w324:bool, element #2=w323:bool)
                n176 = case shown="真" w324 {
                  tunnel: w323 -> [w333 _]
                  tunnel: w322 -> [w332 w347]
                  tunnel: w321 -> [w330 w341]
                  frame False {
                    n177 = Unbundle By Name(w332) -> ("氨氮"=w331:bool)
                    n178 = case shown="真" w333 {
                      tunnel: w331 -> [_ w335]
                      tunnel: w330 -> [_ w334]
                      frame False {
                      }
                      frame True {
                        n179 = case shown="真" w335 {
                          tunnel: w334 -> [_ w336]
                          tunnel: [_ w337] -> _
                          frame False {
                          }
                          frame True {
                            n180 = call "取水点无水样数据存储.vi"("数据标识"="lw", "数据类型"=w336, "table"="氨氮") -> ("error out"=w337:errorcluster)  [unwired: 8 in]
                          }
                        }
                      }
                    }
                  }
                  frame True {
                    n181 = Unbundle By Name(w347) -> ("氨氮"=w346:bool, "CODMn"=w345:bool, "CODcr"=w344:bool, "多参数"=w343:bool, "总氮"=w342:bool, "总磷"=w340:bool)
                    n182 = case shown="真" w346 {
                      tunnel: w341 -> [_ w398]
                      tunnel: [_ w399] -> _
                      frame False {
                      }
                      frame True {
                        n183 = call "取水点无水样数据存储.vi"("数据标识"="Z", "数据类型"=w398, "table"="氨氮") -> ("error out"=w399:errorcluster)  [unwired: 8 in]
                      }
                    }
                    n184 = case shown="真" w342 {
                      tunnel: w341 -> [_ w351]
                      frame False {
                      }
                      frame True {
                        n185 = call "取水点无水样数据存储.vi"("数据标识"="Z", "数据类型"=w351, "table"="总氮") -> ()  [unwired: 8 in, 1 out]
                      }
                    }
                    n186 = case shown="真" w345 {
                      tunnel: w341 -> [_ w395]
                      tunnel: [_ w394] -> _
                      frame False {
                      }
                      frame True {
                        n187 = call "取水点无水样数据存储.vi"("数据标识"="Z", "数据类型"=w395, "table"="CODMn") -> ("error out"=w394:errorcluster)  [unwired: 8 in]
                      }
                    }
                    n188 = case shown="真" w344 {
                      tunnel: w341 -> [_ w391]
                      tunnel: [_ w390] -> _
                      frame False {
                      }
                      frame True {
                        n189 = call "取水点无水样数据存储.vi"("数据标识"="Z", "数据类型"=w391, "table"="CODCr") -> ("error out"=w390:errorcluster)  [unwired: 8 in]
                      }
                    }
                    n190 = case shown="真" w343 {
                      tunnel: w341 -> [_ w361]
                      frame False {
                      }
                      frame True {
                        n191 = global read "断电保存变量.vi" "Cond"() -> (w355:bool)
                        n192 = global read "断电保存变量.vi" "Turb"() -> (w356:bool)
                        n193 = global read "断电保存变量.vi" "DO"() -> (w357:bool)
                        n194 = global read "断电保存变量.vi" "pH"() -> (w358:bool)
                        n195 = global read "断电保存变量.vi" "Temp"() -> (w359:bool)
                        n196 = case shown="真" w358 {
                          tunnel: w361 -> [_ w383]
                          tunnel: [_ w382] -> _
                          frame False {
                          }
                          frame True {
                            n197 = call "取水点无水样数据存储.vi"("数据标识"="Z", "数据类型"=w383, "table"="pH") -> ("error out"=w382:errorcluster)  [unwired: 8 in]
                          }
                        }
                        n198 = case shown="真" w357 {
                          tunnel: w361 -> [_ w379]
                          tunnel: [_ w378] -> _
                          frame False {
                          }
                          frame True {
                            n199 = call "取水点无水样数据存储.vi"("数据标识"="Z", "数据类型"=w379, "table"="DO") -> ("error out"=w378:errorcluster)  [unwired: 8 in]
                          }
                        }
                        n200 = case shown="真" w356 {
                          tunnel: w361 -> [_ w371]
                          tunnel: [_ w370] -> _
                          frame False {
                          }
                          frame True {
                            n201 = call "取水点无水样数据存储.vi"("数据标识"="Z", "数据类型"=w371, "table"="浊度") -> ("error out"=w370:errorcluster)  [unwired: 8 in]
                          }
                        }
                        n202 = case shown="真" w355 {
                          tunnel: w361 -> [_ w375]
                          tunnel: [_ w374] -> _
                          frame False {
                          }
                          frame True {
                            n203 = call "取水点无水样数据存储.vi"("数据标识"="Z", "数据类型"=w375, "table"="比电导率") -> ("error out"=w374:errorcluster)  [unwired: 8 in]
                          }
                        }
                        n204 = case shown="真" FALSE {
                          tunnel: w361 -> [_ w363]
                          tunnel: [_ w362] -> _
                          frame False {
                          }
                          frame True {
                            n205 = call "取水点无水样数据存储.vi"("数据标识"="Z", "数据类型"=w363, "table"="藻密度") -> ("error out"=w362:errorcluster)  [unwired: 8 in]
                          }
                        }
                        n206 = global read "断电保存变量.vi" "叶绿素a启用"() -> (w354:bool)
                        n207 = case shown="真" w359 {
                          tunnel: w361 -> [_ w387]
                          tunnel: [_ w386] -> _
                          frame False {
                          }
                          frame True {
                            n208 = call "取水点无水样数据存储.vi"("数据标识"="Z", "数据类型"=w387, "table"="水温") -> ("error out"=w386:errorcluster)  [unwired: 8 in]
                          }
                        }
                        n209 = case shown="真" w354 {
                          tunnel: w361 -> [_ w367]
                          tunnel: [_ w366] -> _
                          frame False {
                          }
                          frame True {
                            n210 = call "取水点无水样数据存储.vi"("数据标识"="Z", "数据类型"=w367, "table"="叶绿素") -> ("error out"=w366:errorcluster)  [unwired: 8 in]
                          }
                        }
                      }
                    }
                    n211 = case shown="真" w340 {
                      tunnel: [_ w348] -> _
                      frame False {
                      }
                      frame True {
                        n212 = call "取水点无水样数据存储.vi"("数据标识"="Z", "table"="总磷") -> ("error out"=w348:errorcluster)  [unwired: 9 in]
                      }
                    }
                  }
                }
              }
              frame "集成干预" {
                n213 = Unbundle By Name(w408) -> ("总磷"=w402:bool, "总氮"=w403:bool, "氨氮"=w407:bool, "CODMn"=w406:bool, "CODcr"=w405:bool, "多参数"=w404:bool)
                n214 = case shown="真" w402 {
                  frame False {
                  }
                  frame True {
                    n215 = call "获取最近两组水样测试数据.vi"("table"="总磷") -> ("error out"=w414:errorcluster, "存储变量"=w413:T13)  [unwired: 9 in]
                    n216 = call "集成干预测试数据存储.vi"("error in (no error)"=w414, "存储变量"=w413) -> ()  [unwired: 9 in, 1 out]
                  }
                }
                n217 = case shown="真" w403 {
                  frame False {
                  }
                  frame True {
                    n218 = call "获取最近两组水样测试数据.vi"("table"="总氮") -> ("error out"=w411:errorcluster, "存储变量"=w410:T13)  [unwired: 9 in]
                    n219 = call "集成干预测试数据存储.vi"("error in (no error)"=w411, "存储变量"=w410) -> ()  [unwired: 9 in, 1 out]
                  }
                }
                n220 = case shown="真" w407 {
                  frame False {
                  }
                  frame True {
                    n221 = call "获取最近两组水样测试数据.vi"("table"="氨氮") -> ("error out"=w472:errorcluster, "存储变量"=w473:T13)  [unwired: 9 in]
                    n222 = call "集成干预测试数据存储.vi"("error in (no error)"=w472, "存储变量"=w473) -> ("error out"=w468:errorcluster)  [unwired: 9 in]
                    n223 = call "获取最近两组水样测试数据.vi"("error in (no error)"=w468, "table"="总磷") -> ("error out"=w471:errorcluster, "存储变量"=w470:T13)  [unwired: 8 in]
                    n224 = call "集成干预测试数据存储.vi"("error in (no error)"=w471, "存储变量"=w470) -> ()  [unwired: 9 in, 1 out]
                  }
                }
                n225 = case shown="真" w406 {
                  frame False {
                  }
                  frame True {
                    n226 = call "获取最近两组水样测试数据.vi"("table"="CODMn") -> ("error out"=w465:errorcluster, "存储变量"=w466:T13)  [unwired: 9 in]
                    n227 = call "集成干预测试数据存储.vi"("error in (no error)"=w465, "存储变量"=w466) -> ()  [unwired: 9 in, 1 out]
                  }
                }
                n228 = case shown="真" w405 {
                  frame False {
                  }
                  frame True {
                    n229 = call "获取最近两组水样测试数据.vi"("table"="CODCr") -> ("error out"=w462:errorcluster, "存储变量"=w463:T13)  [unwired: 9 in]
                    n230 = call "集成干预测试数据存储.vi"("error in (no error)"=w462, "存储变量"=w463) -> ()  [unwired: 9 in, 1 out]
                  }
                }
                n231 = case shown="真" w404 {
                  frame False {
                  }
                  frame True {
                    n232 = global read "断电保存变量.vi" "Temp"() -> (w421:bool)
                    n233 = case shown="真" w421 {
                      tunnel: [_ w458] -> w427
                      frame False {
                      }
                      frame True {
                        n234 = call "获取最近两组水样测试数据.vi"("table"="水温") -> ("error out"=w461:errorcluster, "存储变量"=w460:T13)  [unwired: 9 in]
                        n235 = call "集成干预测试数据存储.vi"("error in (no error)"=w461, "存储变量"=w460) -> ("error out"=w458:errorcluster)  [unwired: 9 in]
                      }
                    }
                    n236 = global read "断电保存变量.vi" "pH"() -> (w420:bool)
                    n237 = case shown="真" w420 {
                      tunnel: [_ w454] -> w426
                      tunnel: w427 -> [_ w453]
                      frame False {
                      }
                      frame True {
                        n238 = call "获取最近两组水样测试数据.vi"("error in (no error)"=w453, "table"="pH") -> ("error out"=w457:errorcluster, "存储变量"=w456:T13)  [unwired: 8 in]
                        n239 = call "集成干预测试数据存储.vi"("error in (no error)"=w457, "存储变量"=w456) -> ("error out"=w454:errorcluster)  [unwired: 9 in]
                      }
                    }
                    n240 = global read "断电保存变量.vi" "DO"() -> (w419:bool)
                    n241 = case shown="真" w419 {
                      tunnel: [_ w449] -> w425
                      tunnel: w426 -> [_ w448]
                      frame False {
                      }
                      frame True {
                        n242 = call "获取最近两组水样测试数据.vi"("error in (no error)"=w448, "table"="DO") -> ("error out"=w452:errorcluster, "存储变量"=w451:T13)  [unwired: 8 in]
                        n243 = call "集成干预测试数据存储.vi"("error in (no error)"=w452, "存储变量"=w451) -> ("error out"=w449:errorcluster)  [unwired: 9 in]
                      }
                    }
                    n244 = global read "断电保存变量.vi" "Cond"() -> (w418:bool)
                    n245 = case shown="真" w418 {
                      tunnel: [_ w444] -> w424
                      tunnel: w425 -> [_ w443]
                      frame False {
                      }
                      frame True {
                        n246 = call "获取最近两组水样测试数据.vi"("error in (no error)"=w443, "table"="比电导率") -> ("error out"=w447:errorcluster, "存储变量"=w446:T13)  [unwired: 8 in]
                        n247 = call "集成干预测试数据存储.vi"("error in (no error)"=w447, "存储变量"=w446) -> ("error out"=w444:errorcluster)  [unwired: 9 in]
                      }
                    }
                    n248 = global read "断电保存变量.vi" "Turb"() -> (w417:bool)
                    n249 = case shown="真" w417 {
                      tunnel: [_ w439] -> w423
                      tunnel: w424 -> [_ w438]
                      frame False {
                      }
                      frame True {
                        n250 = call "获取最近两组水样测试数据.vi"("error in (no error)"=w438, "table"="浊度") -> ("error out"=w442:errorcluster, "存储变量"=w441:T13)  [unwired: 8 in]
                        n251 = call "集成干预测试数据存储.vi"("error in (no error)"=w442, "存储变量"=w441) -> ("error out"=w439:errorcluster)  [unwired: 9 in]
                      }
                    }
                    n252 = global read "断电保存变量.vi" "叶绿素a启用"() -> (w416:bool)
                    n253 = case shown="真" w416 {
                      tunnel: [_ w434] -> w422
                      tunnel: w423 -> [_ w433]
                      frame False {
                      }
                      frame True {
                        n254 = call "获取最近两组水样测试数据.vi"("error in (no error)"=w433, "table"="叶绿素") -> ("error out"=w437:errorcluster, "存储变量"=w436:T13)  [unwired: 8 in]
                        n255 = call "集成干预测试数据存储.vi"("error in (no error)"=w437, "存储变量"=w436) -> ("error out"=w434:errorcluster)  [unwired: 9 in]
                      }
                    }
                    n256 = case shown="真" FALSE {
                      tunnel: [_ w429] -> _
                      tunnel: w422 -> [_ w428]
                      frame False {
                      }
                      frame True {
                        n257 = call "获取最近两组水样测试数据.vi"("error in (no error)"=w428, "table"="藻密度") -> ("error out"=w432:errorcluster, "存储变量"=w431:T13)  [unwired: 8 in]
                        n258 = call "集成干预测试数据存储.vi"("error in (no error)"=w432, "存储变量"=w431) -> ("error out"=w429:errorcluster)  [unwired: 9 in]
                      }
                    }
                  }
                }
              }
            }
          }
        }
        n259 = global read "采配水全局变量.vi" "状态"() -> (w316:T8)
        n260 = Unbundle By Name(w316) -> ("R0"=w315:i16)
        n261 = Equal To 0?(x=w315) -> (x = 0?=w314:bool)
        n262 = Select(t=enum16{"初始化", "采配水启动", "仪器操作", "反冲洗", "结束"}."结束" ("枚举"), s=w314, f=enum16{"初始化", "采配水启动", "仪器操作", "反冲洗", "结束"}."反冲洗" ("枚举")) -> (s? t:f=w311:enum16{"初始化", "采配水启动", "仪器操作", "反冲洗", "结束"})
      }
      frame "结束" {
        n263 = Release Queue(queue=w479) -> ()  [unwired: 2 in, 3 out]
        n264 = Unbundle By Name(w476) -> ("测试模式"=w477:enum16{"正常测试", "集成干预"})
        n265 = Cancel Notification(0:w480) -> (8:w481:refnum<notifier>)  [unwired: 1 in, 2 out]
        n266 = Release Notifier(notifier=w481) -> ()  [unwired: 2 in, 3 out]
        n267 = case shown="\"集成干预\"" w477 {
          tunnel: w475 -> [_ w484]
          frame "正常测试", Default {
          }
          frame "集成干预" {
            n268 = global write "系统设置全局变量.vi" "运行模式"(w484) -> ()
          }
        }
      }
    }
    n269 = Format Into String(format string="%s,当前运行时间%d秒" ("格式字符串"), w15, w11) -> (resulting string=w16:string)  [unwired: 2 in, 1 out]
    n270 = global write "采配水全局变量.vi" "运行状态显示"(w16) -> ()
  }
